vi "Array of U32_Read.vi"(8 "error in (no error)":errorcluster, 9 "Default":u32[](array[numeric]), 11 "Tag Name":string) -> (0 "error out":errorcluster, 1 "Value":u32[](array[numeric]))   [LabVIEW 2016, in "CVT.lvlib" / "Current Value Table.lvlib"]
doc: "This VI will read the data associated with a single tag. This VI will always look up the tag index if the name changes, or if index lookup failed previously (resulting in an error). This combines the functionality of the CVT2 VIs for reads and static reads."
uses:
  <vilib>/NI/Current Value Table/Current Value Table.lvlib
  <vilib>/NI/Current Value Table/FGVs/Tag Memory Methods.ctl
  <vilib>/NI/Current Value Table/Type Defs/Memory Commands.ctl
  <vilib>/NI/Current Value Table/DataTypes/Array of U32_Type To Enum.vi
  <vilib>/NI/Current Value Table/DataTypes/Array of U32_Memory Block.vi
  <vilib>/NI/Current Value Table/FGVs/CVT Globals.vi
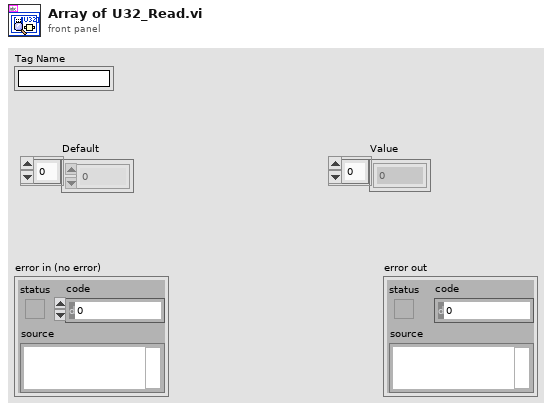
[diagram p1: front panel]
types:
  T1 = typedef "CVT.lvlib/Current Value Table.lvlib/Tag Memory Methods.ctl" = enum16{"Clear", "Read Tag Index", "Read Tag Indices", "Generate Group", "Add Tag", "Overwrite Tag", "Read Description", "Get Stored Tags"}
  T2 = typedef "CVT.lvlib/Current Value Table.lvlib/Data Types.ctl" = enum16{"Double", "Single", "I64", "I32", "I16", "I8", "U64", "U32", "U16", "U8", "String", "Boolean", "Array of U8", "Array of U16", "Array of U32", "Array of U64", "Array of I64", "Array of I32", "Array of I16", "Array of I8", "Array of Double", "Array of Single", "Array of Boolean", "Array of String"}
  T3 = typedef "CVT.lvlib/Current Value Table.lvlib/Memory Commands.ctl" = enum16{"Init", "Add Data", "Read", "Read Group", "Read All", "Write", "Write Group", "Get Size"}
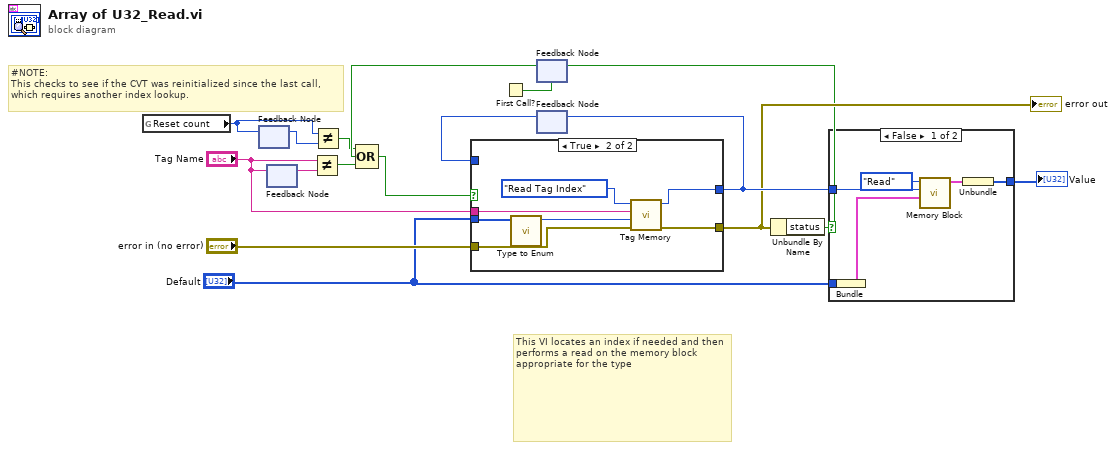
[diagram p0: block diagram]
diagram:
  # "#NOTE:\nThis checks to see if the CVT was reinitialized since the last call,\nwhich requires another index lookup."
  # "This VI locates an index if needed and then performs a read on the memory block appropriate for the type"
  n1 = global read "CVT Globals.vi" "Reset count"() -> (w2:u32)
  n2 = feedback #1() -> (w3:u32)  [unwired: 1 in]
  n3 = feedback-in #1(w2) -> ()
  n4 = feedback #2() -> (w15:string)  [unwired: 1 in]
  n5 = feedback-in #2("Tag Name") -> ()
  n6 = Not Equal?(x="Tag Name", y=w15) -> (x != y?=w10:bool)
  n7 = Not Equal?(x=w2, y=w3) -> (x != y?=w1:bool)
  n8 = First Call?() -> (First Call?: T/F=w6:bool)
  n9 = feedback #3(w6) -> (w8:bool)
  n10 = Compound Arithmetic op=OR(w1, w8, w10) -> (w7:bool)
  n11 = feedback #4() -> (w14:i32)  [unwired: 1 in]
  n12 = case shown="True" w7 {
    tunnel: [w18 w24] -> w11
    tunnel: "error in (no error)" -> [w18 w19]
    tunnel: [w17 w23] -> w13
    tunnel: w14 -> [w17 _]
    tunnel: "Default" -> [_ w25]
    tunnel: "Tag Name" -> [_ w20]
    frame False {
      # "Reuse Index"
    }
    frame True {
      n13 = call-poly <vilib>:"Type to Enum.vi"("U32 Array"=w25) -> ("Data Type Enum"=w22:T2)  [unwired: 10 in]
      n14 = call <vilib>:"Tag Memory.vi"("error in (no error)"=w19, "Expected Type"=w22, "Tag"=w20, "Method"=Tag_Memory_Methods."Read Tag Index") -> ("error out"=w24:errorcluster, "Index Out"=w23:i32)  [unwired: 2 in, 4 out]
    }
  }
  "error out" <- w11
  n15 = feedback-in #4(w13) -> ()
  n16 = Unbundle By Name(w11) -> ("status"=w9:bool)
  n17 = feedback-in #3(w9) -> ()
  n18 = case shown="False" w9 {
    tunnel: w13 -> [w30 _]
    tunnel: "Default" -> [w29 w32]
    tunnel: [w26 w32] -> w4
    frame False {
      n19 = Bundle("Default"=w29) -> (w27:cluster{"Default":u32[]})  [unwired: 1 in]
      n20 = call-poly <vilib>:"Memory Block.vi"("Value"=w27, "Index"=w30, "Method"=Memory_Commands."Read") -> ("Value Out"=w28:cluster{"U32 Array":u32[]})  [unwired: 6 in, 2 out]
      n21 = Unbundle(w28) -> ("U32 Array"=w26:u32[])
    }
    frame True {
    }
  }
  "Value" <- w4
